vi "GetVersion.vi"(8 "error in":errorcluster) -> (0 "error out":errorcluster, 3 "Version":string)   [LabVIEW 2020, in "OpenLvVision_OpenCv.lvlib"]
doc: "Returns library version string.\n\nFor example \"3.4.1-dev\"."
uses:
  OpenLvVision_OpenCv.lvlib
  Dlls/OlvOpenCvWrapper.dll
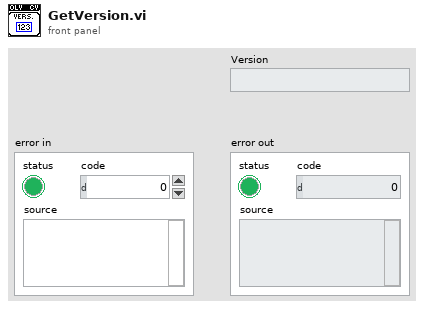
[diagram p1: front panel]
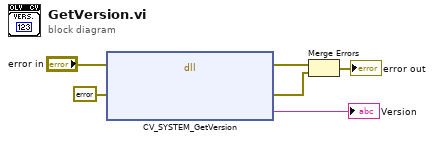
[diagram p0: block diagram]
diagram:
  n1 = dll-call lib="C:/Users/lukas/Downloads/OpenLvVision_OpenCv/SourceCode/LabView/OpenLvVision_OpenCv/Dlls/OlvOpenCvWrapper.dll" fn="CV_SYSTEM_GetVersion"(error in="error in", "Error"=errorcluster {"status"=FALSE, "code"=0, "source"=""} ("error in")) -> (error out=w3:errorcluster, "Error"=w1:errorcluster, "VersionString"=→"Version":string)  [unwired: 4 in, 1 out]
  n2 = Merge Errors(w3, w1) -> (→"error out":errorcluster)
